vi "main.vi"() -> ()   [LabVIEW 2023]
uses:
  #typedef_state.ctl
  #typedef_action.ctl
  #typedef_data.ctl
panel:
  out "Current Defined Steps":dbl[][](array[numeric])
  out "Speed":dbl
  out "Time":dbl
  in  "Slower":bool
  in  "Faster":bool
  in  "Exit":bool
  in  "Define Program":bool
  in  "Start Program":bool
  in  "Quick Start":bool
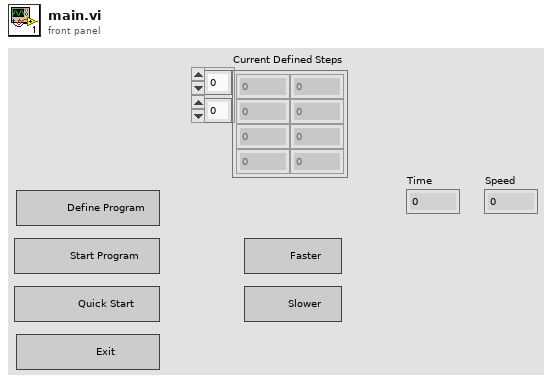
[diagram p1: front panel]
types:
  T1 = typedef "#typedef_state.ctl" = enum16{"Free run", "Staged run", "Defining", "Inicializing"}
  T2 = typedef "#typedef_action.ctl" = enum16{"Run", "Reset"}
  T3 = typedef "#typedef_data.ctl" = cluster{"Current Speed":dbl, "Current Time ":dbl, "reseted?":bool, "Steps":dbl[][], "Time to match":dbl}
  T4 = enum8{"Enabled", "Disabled", "Disabled and Grayed Out"}
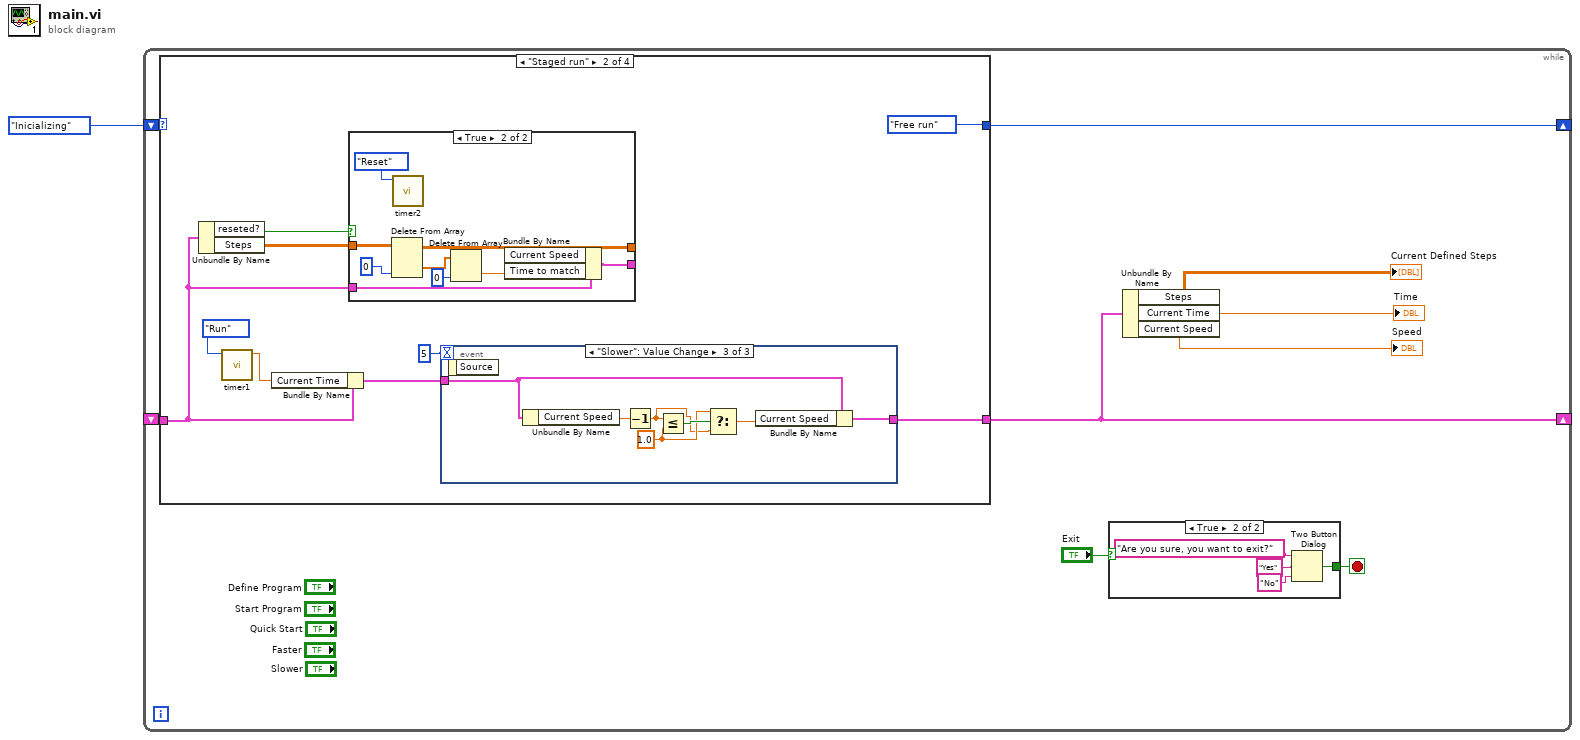
[diagram p0: block diagram]
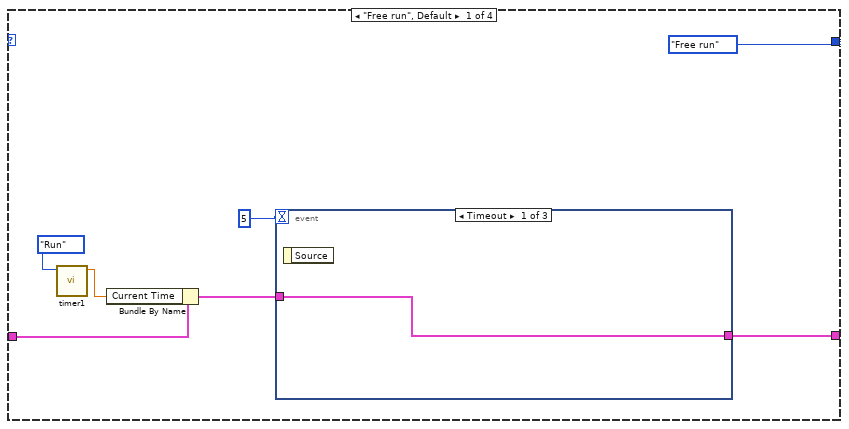
[diagram p2: hidden frame]
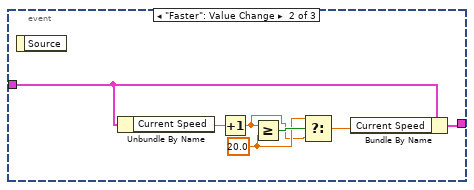
[diagram p3: hidden frame]
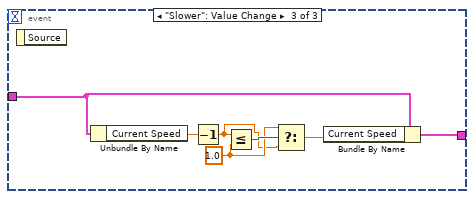
[diagram p4: hidden frame]
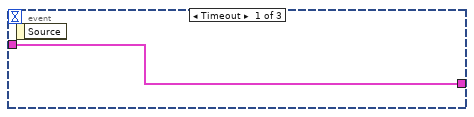
[diagram p6: hidden frame]
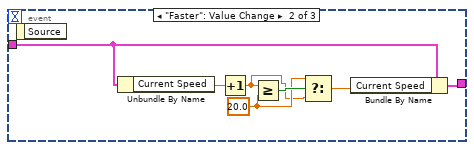
[diagram p7: hidden frame]
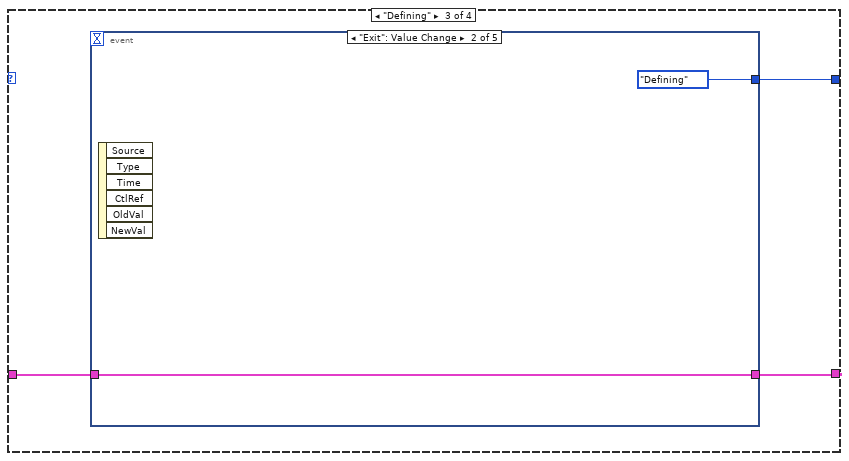
[diagram p8: hidden frame]
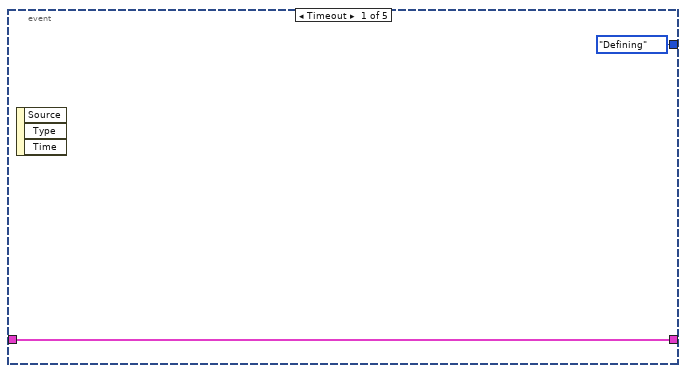
[diagram p9: hidden frame]
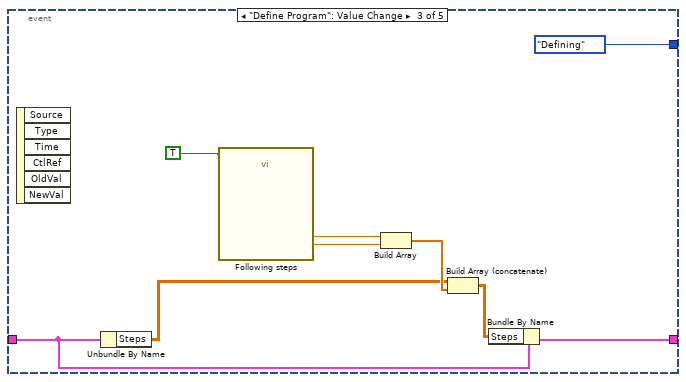
[diagram p10: hidden frame]
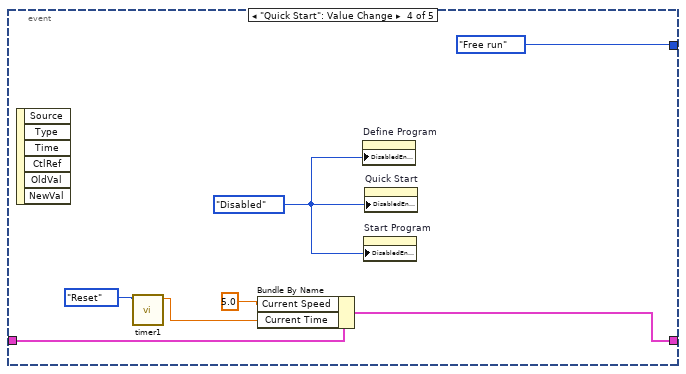
[diagram p11: hidden frame]
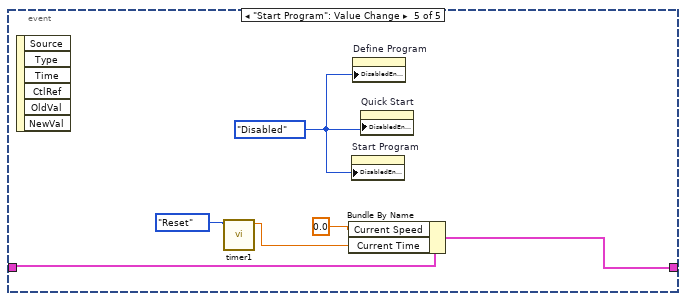
[diagram p12: hidden frame]
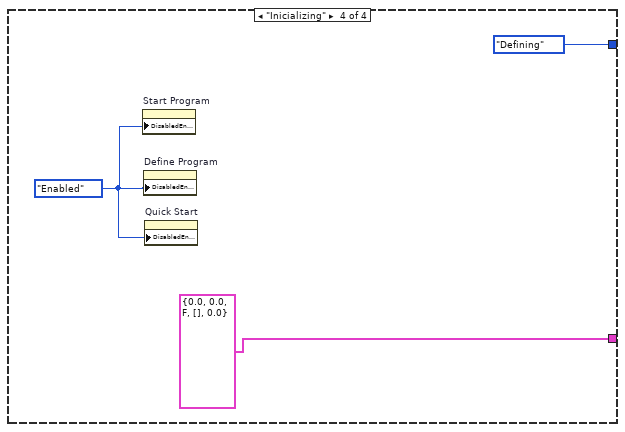
[diagram p13: hidden frame]
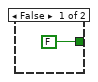
[diagram p14: hidden frame]
diagram:
  n1 = while {
    shift-right: [w7] -> _
    shift-left: #typedef_state."Inicializing" ("State") -> [w8]
    shift-right: [w5] -> _
    shift-left: _ -> [w6]
    stop <- w9 stop-if-true
    n2 = case shown="\"Staged run\"" w8 {
      tunnel: [#typedef_state."Free run" ("State") #typedef_state."Free run" ("State") w67 #typedef_state."Defining" ("State")] -> w7
      tunnel: [w13 w38 w68 T3 {"Current Speed"=0.0, "Current Time "=0.0, "reseted?"=FALSE, "Steps"=[], "Time to match"=0.0} ("Data")] -> w5
      tunnel: w6 -> [w16 w33 w69 _]
      frame "Free run", Default {
        n3 = call "timer1.vi"("Action"=#typedef_action."Run") -> ("Numeric"=w15:dbl)  [unwired: 9 in, 1 out]
        n4 = Bundle By Name(cluster=w16, "Current Time"=w15) -> (w12:T3)
        n5 = event shown="[0] Timeout" {
          selector: _ -> [_ _ _]
          dyn-events: _ -> [_ _ _]
          timeout: 5 -> [_ _ _]
          tunnel: [w18 w19 w26] -> w13
          tunnel: w12 -> [w18 w25 w27]
          event Timeout {
            n6 = event-data() -> ()  [unwired: 1 in, 1 out]
          }
          event "Faster": Value Change {
            w21 = 20.0 ("y")
            n7 = event-data() -> ()  [unwired: 1 in, 1 out]
            n8 = Unbundle By Name(w25) -> ("Current Speed"=w24:dbl)
            n9 = Increment(x=w24) -> (x+1=w20:dbl)
            n10 = Greater Or Equal?(x=w20, y=w21) -> (x >= y?=w23:bool)
            n11 = Select(t=w21, s=w23, f=w20) -> (s? t:f=w22:dbl)
            n12 = Bundle By Name(cluster=w25, "Current Speed"=w22) -> (w19:T3)
          }
          event "Slower": Value Change {
            w29 = 1.0 ("y")
            n13 = event-data() -> ()  [unwired: 1 in, 1 out]
            n14 = Unbundle By Name(w27) -> ("Current Speed"=w32:dbl)
            n15 = Decrement(x=w32) -> (x-1=w28:dbl)
            n16 = Less Or Equal?(x=w28, y=w29) -> (x <= y?=w31:bool)
            n17 = Select(t=w29, s=w31, f=w28) -> (s? t:f=w30:dbl)
            n18 = Bundle By Name(cluster=w27, "Current Speed"=w30) -> (w26:T3)
          }
        }
      }
      frame "Staged run" {
        n19 = Unbundle By Name(w33) -> ("reseted?"=w34:bool, "Steps"=w35:dbl[][])
        n20 = call "timer1.vi"("Action"=#typedef_action."Run") -> ("Numeric"=w41:dbl)  [unwired: 9 in, 1 out]
        n21 = Bundle By Name(cluster=w33, "Current Time"=w41) -> (w39:T3)
        n22 = case shown="True" w34 {
          tunnel: w35 -> [w42 w51]
          tunnel: [w42 w49] -> _
          tunnel: w33 -> [_ w48]
          tunnel: [_ w43] -> _
          frame False {
          }
          frame True {
            n23 = Delete From Array(array=w51, index (col)=0 ("index (row)")) -> (deleted portion=w46:dbl[], array with subset deleted=w49:dbl[][])  [unwired: 2 in]
            n24 = call "timer2.vi"("Action"=#typedef_action."Reset") -> ()  [unwired: 9 in, 2 out]
            n25 = Delete From Array(array=w46, index=0) -> (deleted portion=w47:dbl)  [unwired: 1 in, 1 out]
            n26 = Bundle By Name(cluster=w48, "Time to match"=w47) -> (w43:T3)  [unwired: 1 in]
          }
        }
        n27 = event shown="[2] \"Slower\": Value Change" {
          selector: _ -> [_ _ _]
          dyn-events: _ -> [_ _ _]
          timeout: 5 -> [_ _ _]
          tunnel: [w52 w53 w60] -> w38
          tunnel: w39 -> [w52 w59 w61]
          event Timeout {
            n28 = event-data() -> ()  [unwired: 1 in, 1 out]
          }
          event "Faster": Value Change {
            w55 = 20.0 ("y")
            n29 = event-data() -> ()  [unwired: 1 in, 1 out]
            n30 = Unbundle By Name(w59) -> ("Current Speed"=w58:dbl)
            n31 = Increment(x=w58) -> (x+1=w54:dbl)
            n32 = Greater Or Equal?(x=w54, y=w55) -> (x >= y?=w57:bool)
            n33 = Select(t=w55, s=w57, f=w54) -> (s? t:f=w56:dbl)
            n34 = Bundle By Name(cluster=w59, "Current Speed"=w56) -> (w53:T3)
          }
          event "Slower": Value Change {
            w63 = 1.0 ("y")
            n35 = event-data() -> ()  [unwired: 1 in, 1 out]
            n36 = Unbundle By Name(w61) -> ("Current Speed"=w66:dbl)
            n37 = Decrement(x=w66) -> (x-1=w62:dbl)
            n38 = Less Or Equal?(x=w62, y=w63) -> (x <= y?=w65:bool)
            n39 = Select(t=w63, s=w65, f=w62) -> (s? t:f=w64:dbl)
            n40 = Bundle By Name(cluster=w61, "Current Speed"=w64) -> (w60:T3)
          }
        }
      }
      frame "Defining" {
        n41 = event shown="[1] \"Exit\": Value Change" {
          selector: _ -> [_ _ _ _ _]
          dyn-events: _ -> [_ _ _ _ _]
          timeout: _ -> [_ _ _ _ _]
          tunnel: w69 -> [w71 w73 w77 w88 w92]
          tunnel: [w71 w73 w75 w87 w91] -> w68
          tunnel: [#typedef_state."Defining" ("State") #typedef_state."Defining" ("State") #typedef_state."Defining" ("State") #typedef_state."Free run" ("State") _] -> w67
          event Timeout {
            n42 = event-data() -> ()  [unwired: 1 in, 3 out]
          }
          event "Exit": Value Change {
            n43 = event-data() -> ()  [unwired: 1 in, 6 out]
          }
          event "Define Program": Value Change {
            n44 = event-data() -> ()  [unwired: 1 in, 6 out]
            n45 = Unbundle By Name(w77) -> ("Steps"=w78:dbl[][])
            n46 = call "Following steps"("Enable"=TRUE) -> ("Speed"=w82:dbl, "Time"=w81:dbl)  [unwired: 15 in, 2 out]
            n47 = Build Array(w81, w82) -> (w79:dbl[])
            n48 = Build Array (concatenate)(w78, w79) -> (w76:dbl[][])
            n49 = Bundle By Name(cluster=w77, "Steps"=w76) -> (w75:T3)
          }
          event "Quick Start": Value Change {
            w83 = T4."Disabled" ("Disabled")
            n50 = event-data() -> ()  [unwired: 1 in, 6 out]
            n51 = call "timer1.vi"("Action"=#typedef_action."Reset") -> ("Numeric"=w85:dbl)  [unwired: 9 in, 1 out]
            n52 = Bundle By Name(cluster=w88, "Current Speed"=5.0, "Current Time"=w85) -> (w87:T3)
            n53 = property on="Define Program" class="Bool"("DisabledEnum"=w83) -> ()  [unwired: 2 in, 2 out]
            n54 = property on="Start Program" class="Bool"("DisabledEnum"=w83) -> ()  [unwired: 2 in, 2 out]
            n55 = property on="Quick Start" class="Bool"("DisabledEnum"=w83) -> ()  [unwired: 2 in, 2 out]
          }
          event "Start Program": Value Change {
            w90 = T4."Disabled" ("Disabled")
            n56 = event-data() -> ()  [unwired: 1 in, 6 out]
            n57 = call "timer1.vi"("Action"=#typedef_action."Reset") -> ("Numeric"=w94:dbl)  [unwired: 9 in, 1 out]
            n58 = Bundle By Name(cluster=w92, "Current Speed"=0.0, "Current Time"=w94) -> (w91:T3)
            n59 = property on="Start Program" class="Bool"("DisabledEnum"=w90) -> ()  [unwired: 2 in, 2 out]
            n60 = property on="Define Program" class="Bool"("DisabledEnum"=w90) -> ()  [unwired: 2 in, 2 out]
            n61 = property on="Quick Start" class="Bool"("DisabledEnum"=w90) -> ()  [unwired: 2 in, 2 out]
          }
        }
      }
      frame "Inicializing" {
        w96 = T4."Enabled" ("Disabled")
        n62 = property on="Start Program" class="Bool"("DisabledEnum"=w96) -> ()  [unwired: 2 in, 2 out]
        n63 = property on="Define Program" class="Bool"("DisabledEnum"=w96) -> ()  [unwired: 2 in, 2 out]
        n64 = property on="Quick Start" class="Bool"("DisabledEnum"=w96) -> ()  [unwired: 2 in, 2 out]
      }
    }
    n65 = case shown="True" "Exit" {
      tunnel: [FALSE w103] -> w9
      frame False {
      }
      frame True {
        n66 = Two Button Dialog(message="Are you sure, you want to exit?", 1:"No" ("F button name (\"Cancel\")"), 2:"Yes" ("T button name (\"OK\")")) -> (T button?=w103:bool)
      }
    }
    n67 = Unbundle By Name(w5) -> ("Steps"=→"Current Defined Steps":dbl[][], "Current Time"=→"Time":dbl, "Current Speed"=→"Speed":dbl)
  }
